vi "From Serial Form.vi"(6 "Serial Version":T1, 10 "Deserializer in":refnum<class "Deserializer.lvclass">, 11 "M data in":refnum<class "M data.lvclass">) -> (0 "error out":errorcluster, 2 "Deserializer out":refnum<class "Deserializer.lvclass">, 3 "M data out":refnum<class "M data.lvclass">)   [LabVIEW 2014, in "M data.lvclass"]
uses:
  M data.lvclass
  <vilib>/NI/AQ Character Lineator/Deserializer/Deserializer.lvclass
  <vilib>/NI/AQ Character Lineator/Serialization Common/Serial Version.ctl
  <vilib>/NI/AQ Character Lineator/Serializable/Remove Single.vi
  Alicat Data.lvclass
  <vilib>/NI/AQ Character Lineator/Serializable/Serializable.lvclass
  <vilib>/NI/AQ Character Lineator/Serialization Common/Serialization Common.lvlib
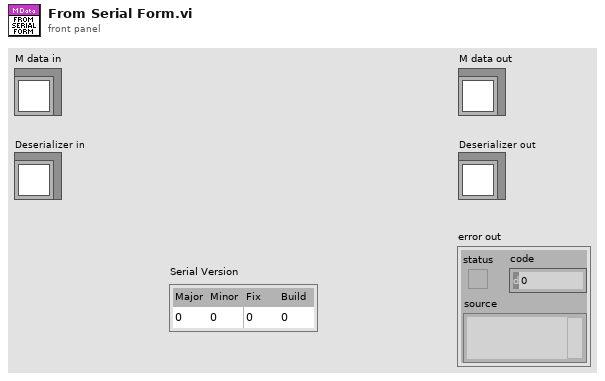
[diagram p1: front panel]
types:
  T1 = typedef "Serialization Common.lvlib/Serial Version.ctl" = cluster{"Major":u16, "Minor":u16, "Fix":u16, "Build":u16}
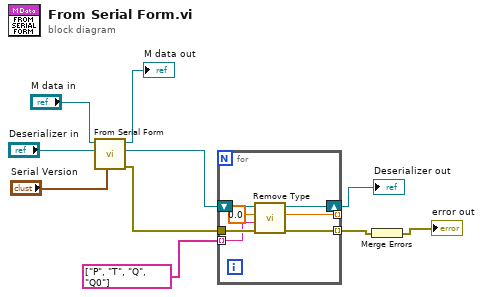
[diagram p0: block diagram]
diagram:
  n1 = call-parent "From Serial Form.vi"("Serial Version"="Serial Version", "Deserializer in"="Deserializer in", "Data in"="M data in") -> ("error out"=w6:errorcluster, "Deserializer out"=w5:refnum<class "Deserializer.lvclass">, "Data out"=→"M data out":refnum<class "M data.lvclass">)  [unwired: 6 in]
  n2 = for {
    tunnel: w6 -> [w17]
    tunnel: string[] ["P", "T", "Q", "Q0"] -> [w15] mode=indexing
    tunnel: [w13] -> _ mode=indexing
    shift-right: [w12] -> w1
    shift-left: w5 -> [w16]
    tunnel: [w11] -> w3 mode=indexing
    n3 = call-poly <vilib>:"Remove Type.vi"("error in (no error)"=w17, "Name"=w15, "Default Value"=sgl 0.0, "Deserializer in"=w16) -> ("error out"=w11:errorcluster, "Numeric"=w13:sgl, "Deserializer out"=w12:refnum<class "Deserializer.lvclass">)  [unwired: 4 in, 1 out]
  }
  "Deserializer out" <- w1
  n4 = Merge Errors(w3) -> (→"error out":errorcluster)
